vi "Check Name Channel Enable.vi"(8 "error in (no error)":errorcluster, 11 "Scan Data Process in":T1) -> (0 "error out":errorcluster, 3 "Scan Data Process out":T1)   [LabVIEW 2015, in "Exposure Process.lvlib"]
uses:
  Exposure Process.lvlib
  Control_Scan Data Process.ctl
  <vilib>/addons/PointValueMap/controls/PointMap.ctl
  Control_EXP Information.ctl
  Control_File Save Setup.ctl
  Control_Enable and Path.ctl
  Control_ICM Export Setting.ctl
  <vilib>/addons/PointValueMap/PointValueMap.lvlib
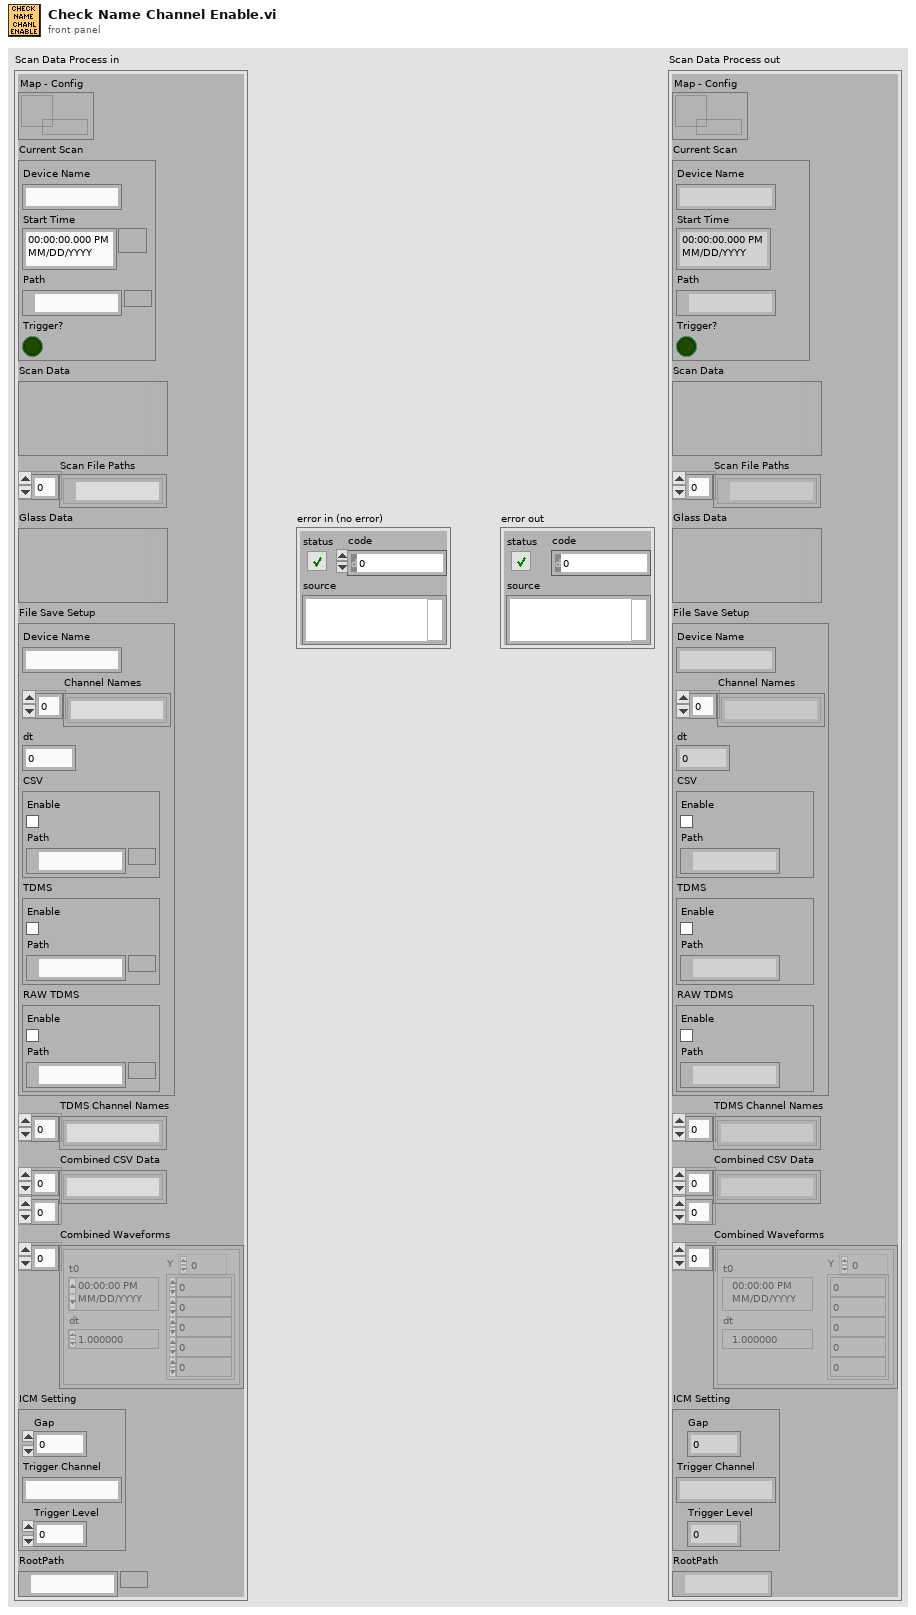
[diagram p1: front panel]
types:
  T1 = typedef "Exposure Process.lvlib/Control_Scan Data Process.ctl" = cluster{"Map - Config":T2, "Current Scan":T3, "Scan Data":variant, "Scan File Paths":path[], "Glass Data":variant, "File Save Setup":T4, "TDMS Channel Names":string[], "Combined CSV Data":string[][], "Combined Waveforms":waveform(dbl)[], "ICM Setting":T6, "RootPath":path}
  T2 = typedef "PointValueMap.lvlib/PointMap.ctl" = refnum<data-value>
  T3 = typedef "Exposure Process.lvlib/Control_EXP Information.ctl" = cluster{"Device Name":string, "Start Time":timestamp, "Path":path, "Trigger?":bool}
  T4 = typedef "Exposure Process.lvlib/Control_File Save Setup.ctl" = cluster{"Device Name":string, "Channel Names":string[], "dt":dbl, "CSV":T5, "TDMS":T5, "RAW TDMS":T5}
  T5 = typedef "Exposure Process.lvlib/Control_Enable and Path.ctl" = cluster{"Enable":bool, "Path":path}
  T6 = typedef "Exposure Process.lvlib/Control_ICM Export Setting.ctl" = cluster{"Gap":dbl, "Trigger Channel":string, "Trigger Level":dbl}
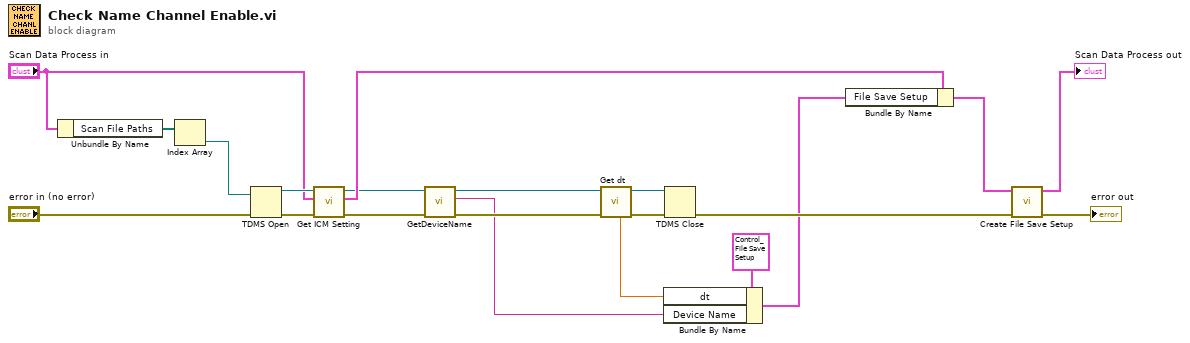
[diagram p0: block diagram]
diagram:
  n1 = Unbundle By Name("Scan Data Process in") -> ("Scan File Paths"=w14:path[])
  n2 = Index Array(array=w14) -> (element=w18:path)  [unwired: 1 in]
  n3 = TDMS Open(8:"error in (no error)", 11:w18) -> (0:w8:errorcluster, 3:w9:refnum<k34>)  [unwired: 5 in]
  n4 = call "Get ICM Setting.vi"("error in (no error)"=w8, "Scan Data Process in"="Scan Data Process in", "tdms file"=w9) -> ("error out"=w4:errorcluster, "Scan Data Process out"=w6:T1, "tdms file out"=w5:refnum<k34>)  [unwired: 5 in, 1 out]
  n5 = call "GetDeviceName.vi"("error in (no error)"=w4, "tdms file"=w5) -> ("error out"=w2:errorcluster, "Device Name"=w1:string, "tdms file out"=w3:refnum<k34>)  [unwired: 7 in]
  n6 = call "Get dt.vi"("error in (no error)"=w2, "tdms file"=w3) -> ("error out"=w20:errorcluster, "tdms file out"=w21:refnum<k34>, "dt"=w16:dbl)  [unwired: 7 in]
  n7 = Bundle By Name(cluster=T4 {"Device Name"="", "Channel Names"=[], "dt"=0.0, "CSV"={"Enable"=FALSE, "Path"=path ""}, "TDMS"={"Enable"=FALSE, "Path"=path ""}, "RAW TDMS"={"Enable"=FALSE, "Path"=path ""}} ("File Save Setup"), "dt"=w16, "Device Name"=w1) -> (w13:T4)
  n8 = TDMS Close(8:w20, 11:w21) -> (0:w15:errorcluster)  [unwired: 1 out]
  n9 = Bundle By Name(cluster=w6, "File Save Setup"=w13) -> (w12:T1)
  n10 = call "Create File Save Setup.vi"("error in (no error)"=w15, "Scan Data Process in"=w12) -> ("error out"=→"error out":errorcluster, "Scan Data Process out"=→"Scan Data Process out":T1)  [unwired: 8 in]
